vi "EventFinderV1.vi"() -> ()   [LabVIEW 2013]
uses:
  <vilib>/Analysis/baseanly.llb/Mean (DBL).vi
  <vilib>/Analysis/5stat.llb/RMS (DBL).vi
  <vilib>/Utility/file.llb/Write To Spreadsheet File (DBL).vi
  <vilib>/Analysis/NI_AALPro.lvlib
  <vilib>/Analysis/NI_AALBase.lvlib
panel:
  in  "Points":i32=2
  in  "Median filter":bool
  in  "Reverse trace in time":bool
  in  "Reduce points to display by factor":i32=10
  out "?":bool=TRUE
  in  "Peak over DNA level/nA":dbl=-0.05
  out "?":bool=TRUE
  in  "DNA level/nA":dbl=-0.1
  out "?":bool=TRUE
  in  "21 over DNA level/nA":dbl=-0.02
  in  "Each event as separate file":bool
  in  "Custom dt":cluster{"Custom dt":dbl, "Custom dt":bool}={"Custom dt"=4e-06, "Custom dt"=FALSE}
  in  "Fraction from start":dbl=0.1
  in  "Type 21 limit":bool
  in  "Baseline correction":T1={"Baseline correction?"=TRUE, "Correction method"=enum."Median", "Points for \nbaseline "=125000, "Value  if \nsubtracting"=0.0, "Order if using polynomial"=3, "Use file \nlength"=TRUE}
  in  "Output folder name":string="Output"
  in  "Loop over \nfolder of folders":bool
  in  "Directory of subfolders":path=path "F:/"
  out "Cumulative time/s":dbl=1130.5142
  out "File mean":dbl=-0.4359130217142997 format="%0.2f"
  out "File RMS":dbl=12.404886152154484 format="%0.4f"
  out "Cumulative time/s":dbl=1429.5900000000001
  in  "Numbers off":bool
  in  "Move this file to \n\"noise\" folder":bool
  in  "Graphs off":bool
  in  "Limit in peak current":bool
  in  "Invert trace":bool
  in  "Event begin+end/nA":dbl=-0.06
  in  "Each event in separate column":bool
  in  "Events concatenated into one column":bool
  in  "More than/fAs":dbl=50.0
  in  "Less than/fAs":dbl=500.0
  in  "Limit in area":bool
  out "Raw current":waveform(dbl)(graph)={"t0"=timestamp(0 s since 1904-01-01), "dt"=0.0002, "Y"=[]}
  in  "Pause at new file?":bool
  in  "Finish here":bool
  in  "Jump file":bool
  out "Time since last/s":dbl=0.2605 format="%0.5f"
  out "Time in file/s":dbl=0.9242 format="%0.3f"
  in  "Reject on":bool
  out "Duration/s":dbl=0.0009600000000000003 format="%0.5f"
  out "Mean current/nA":dbl=-108.25728329022725 format="%0.5f"
  out "Peak value/nA":dbl=-147.76609802246094 format="%0.5f"
  out "Event area/fAs":dbl=103839.10133361818 format="%0.5f"
  out "dt/s":dbl=2e-05
  in  "Event statistics":bool=TRUE
  out "Accepted events":i32=475
  in  "Reject":bool
  in  "Loop delay/s":dbl
  out "Current file":i32=5
  out "Current file name":path
  out "No files":i32=7
  in  "Directory of files":path=path "C:/"
  out "Event detection trace":waveform(dbl)(graph)={"t0"=timestamp(0 s since 1904-01-01), "dt"=2e-05, "Y"=[]}
  in  "Accept on":bool
  out "Current trace after filter, baseline correction":waveform(dbl)(graph)={"t0"=timestamp(0 s since 1904-01-01), "dt"=0.0002, "Y"=[]}
  in  "Accept":bool
  in  "Points before/after":i32=50
  in  "Min duration/s":dbl=0.0005
  in  "Threshold/nA":dbl=-0.1
  # "Event detection settings"
  # "Files to save"
  # "Data input settings"
  # "Limit in event area"
  # "Event stats"
  # "Speed up\n analysis"
  # "Slow analysis \nfor viewing"
  # "Actions"
  # "Further data input settings"
  # "Limit according to DNA level"
  # "Set DNA level:"
  # "Use files in multiple folders"
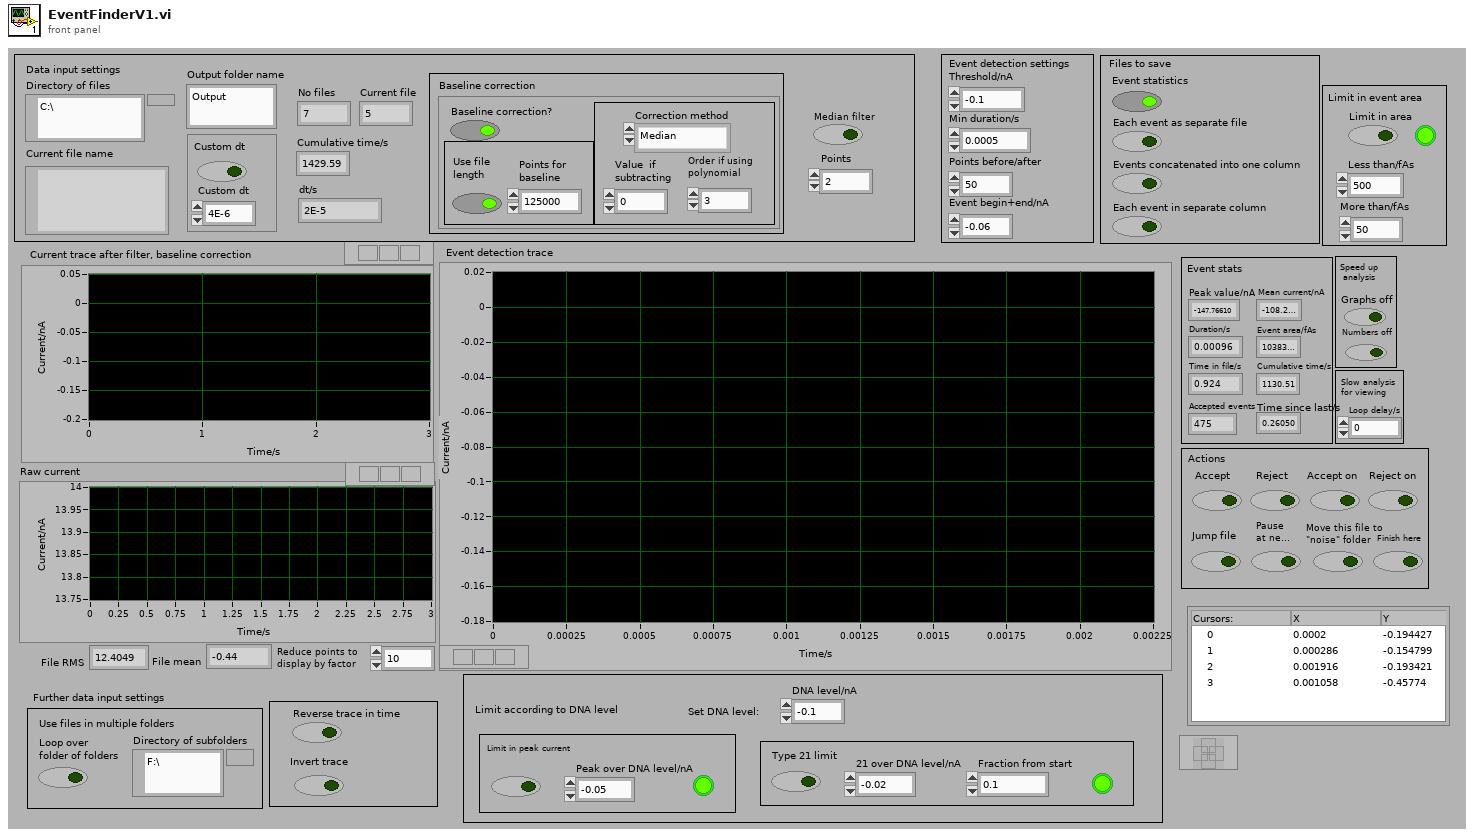
[diagram p1: front panel]
types:
  T1 = cluster{"Baseline correction?":bool, "Correction method":enum16{"Linear", "Median", "Mean", "Polynomial", "Subtraction"}, "Points for \nbaseline ":i32, "Value  if \nsubtracting":dbl, "Order if using polynomial":i32, "Use file \nlength":bool}
  T2 = enum16{"Linear", "Median", "Mean", "Polynomial", "Subtraction"}
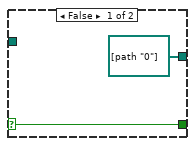
[diagram p2: hidden frame]
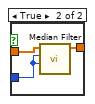
[diagram p7: hidden frame]
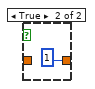
[diagram p8: hidden frame]
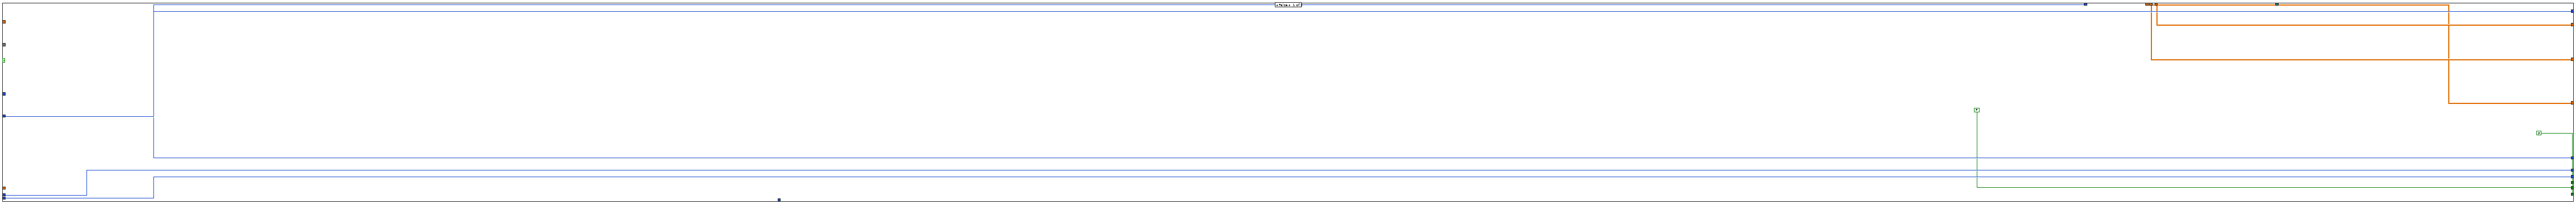
[diagram p15: hidden frame]
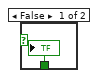
[diagram p18: hidden frame]
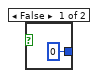
[diagram p20: hidden frame]
diagram:
  n1 = case shown="True" "Loop over \nfolder of folders" {
    selector: "Loop over \nfolder of folders" -> [w5 w7]
    tunnel: "Directory of subfolders" -> [_ w10]
    tunnel: [path[] [path "0"] w9] -> w4
    tunnel: [w5 w7] -> w3
    frame False {
    }
    frame True {
      n2 = List Folder(path=w10) -> (folder names=w8:string[])  [unwired: 1 in, 5 out]
      n3 = for {
        tunnel: w10 -> [w13]
        tunnel: [w12] -> w9 mode=indexing
        tunnel: w8 -> [w11] mode=indexing
        n4 = Build Path(base path=w13, name or relative path=w11) -> (appended path=w12:path)
      }
    }
  }
  n5 = for {
    tunnel: w4 -> [w33] mode=indexing
    tunnel: w3 -> [w21]
    # "Initialize arrays"
    # "Loop over folders if selected"
    n6 = case shown="False" w21 {
      tunnel: ["Directory of files" w72] -> w69
      tunnel: w33 -> [_ w72]
      frame False {
      }
      frame True {
      }
    }
    n7 = Initialize Array(0.0 ("element"), 0 ("dimension size"), 0 ("dimension size")) -> (w58:dbl[][])
    n8 = call "Make output folder.vi"("Output folder name"="Output folder name", "Folder"=w69) -> ("created path"=w68:path)
    n9 = call "Create array of files in folder.vi"("Folder"=w69) -> ("No files"=→"No files":i32, "Array of files in folder"=w14:path[])  [unwired: 1 in]
    n10 = Initialize Array(0.0 ("element"), 0 ("dimension size"), 0 ("dimension size")) -> (w53:dbl[][])
    n11 = Initialize Array(0.0 ("element"), 0 ("dimension size"), 0 ("dimension size")) -> (w64:dbl[][])
    n12 = for {
      tunnel: w14 -> [w101] mode=indexing
      tunnel: w68 -> [w99]
      shift-right: [w125] -> w36
      shift-left: w64 -> [w130]
      tunnel: [w91] -> w44
      shift-right: [w128] -> _
      shift-left: 0 -> [w129]
      shift-right: [w120] -> w57
      shift-left: w58 -> [w121]
      shift-right: [w118] -> w42
      shift-left: w53 -> [w119]
      shift-right: [w105] -> w28
      shift-left: 0 -> [w113]
      shift-right: [w106] -> _
      shift-left: 0.0 -> [w107]
      i -> [w131]
      stop <- w124 stop-if-true
      # "Loop over files in folder"
      n13 = Increment(x=w131) -> (x+1=w122:i32)
      "Current file" <- w122
      n14 = case shown="True" "Pause at new file?" {
        frame False {
        }
        frame True {
          n15 = property on="Reject on" class="Bool (strict)"("Value"=FALSE ("Keep rejecting")) -> ()  [unwired: 2 in, 2 out]
          n16 = property on="Accept on" class="Bool (strict)"("Value"=FALSE ("Keep accepting")) -> ()  [unwired: 2 in, 2 out]
        }
      }
      n17 = call "Baselinecorrector.vi"("Custom dt"="Custom dt", "Path"=w101, "Baseline param"="Baseline correction") -> ("Raw current"=w103:waveform(dbl), "Filtered, baseline corrected"=w89:dbl[], "dt"=w92:dbl)  [unwired: 3 in, 1 out]
      n18 = case shown="False" "Median filter" {
        tunnel: w89 -> [w133 w136]
        tunnel: "Points" -> [_ w135]
        tunnel: [w133 w134] -> w87
        frame False {
        }
        frame True {
          n19 = call <vilib>:"Median Filter.vi"("right rank"=w135, "left rank"=w135, "X"=w136) -> ("Filtered X"=w134:dbl[])  [unwired: 7 in, 1 out]
        }
      }
      n20 = case shown="True" "Reverse trace in time" {
        tunnel: w87 -> [w142 w144]
        tunnel: [w142 w143] -> w117
        frame False {
        }
        frame True {
          n21 = Reverse 1D Array(array=w144) -> (reversed array=w143:dbl[])
        }
      }
      n22 = case shown="True" "Invert trace" {
        tunnel: w117 -> [w139 w141]
        tunnel: [w139 w140] -> w102
        frame False {
        }
        frame True {
          n23 = Negate(x=w141) -> (-x=w140:dbl[])
        }
      }
      n24 = Array Size(array=w102) -> (size(s)=w97:i32)
      n25 = Add(x=w97, y=w113) -> (x+y=w112:i32)
      n26 = call-poly <vilib>:"Mean.vi"("X"=w102) -> ("mean"=→"File mean":dbl)  [unwired: 1 out]
      n27 = call-poly <vilib>:"RMS.vi"("X"=w102) -> ("rms value"=→"File RMS":dbl)  [unwired: 1 out]
      n28 = Bundle By Name("dt"=w92, "Y"=w102) -> (w114:waveform(dbl))  [unwired: 1 out]
      n29 = Equal To 0?(x=w92) -> (x = 0?=w110:bool)
      n30 = case shown="False" w110 {
        tunnel: [w137 1] -> w111
        tunnel: w92 -> [w137 _]
        frame False {
        }
        frame True {
        }
      }
      "dt/s" <- w111
      n31 = local read "Graphs off"() -> (w115:bool)
      n32 = call "Display traces.vi"("Graphs off"=w115, "Raw current in"=w103, "Display reduction"="Reduce points to display by factor", "Waveform"=w114) -> ("Raw current out"=→"Raw current":waveform(dbl), "Baseline corrected current trace"=→"Current trace after filter, baseline correction":waveform(dbl))  [unwired: 6 in]
      n33 = while {
        tunnel: w102 -> [w178]
        shift-right: [w180] -> _
        shift-left: 0 -> [w181]
        tunnel: w111 -> [w149]
        tunnel: w97 -> [w147]
        shift-right: [w166] -> w125
        shift-left: w130 -> [w177]
        shift-right: [w154] -> w128
        shift-left: w129 -> [w176]
        shift-right: [w175] -> _
        shift-left: 0 -> [w174]
        shift-right: [w171] -> _
        shift-left: 0 -> [w172]
        tunnel: [w167] -> w124
        tunnel: w122 -> [w165]
        shift-right: [w164] -> w120
        shift-left: w121 -> [w163]
        shift-right: [w161] -> w118
        shift-left: w119 -> [w162]
        tunnel: w112 -> [w153]
        tunnel: [w153] -> w105
        tunnel: w107 -> [w152]
        tunnel: [w149] -> w104
        tunnel: w99 -> [w148]
        tunnel: [w148] -> w91
        stop <- w168 stop-if-true
        # "While loop through file to search for events"
        n34 = Greater Or Equal?(x=w181, y=w147) -> (x >= y?=w169:bool)
        n35 = Increment(x=w181) -> (x+1=w179:i32)
        n36 = Index Array(array=w178, index=w179) -> (element=w160:dbl)
        n37 = Less?(x=w160, y="Threshold/nA") -> (x < y?=w159:bool)
        n38 = Multiply(x=w153, y=w149) -> (x*y=→"Cumulative time/s":dbl)
        n39 = case shown="True" w159 {
          tunnel: w178 -> [_ w249]
          tunnel: w179 -> [w203 w212]
          tunnel: [w203 w221] -> w180
          tunnel: "Points before/after" -> [_ w220]
          tunnel: w149 -> [_ w214]
          tunnel: [w202 w245] -> w166
          tunnel: w177 -> [w202 w215]
          tunnel: w176 -> [w201 w244]
          tunnel: [w201 w243] -> w154
          tunnel: [w200 w242] -> w175
          tunnel: w174 -> [w200 w207]
          tunnel: w172 -> [w199 w237]
          tunnel: [w199 w238] -> w171
          tunnel: [w195 w236] -> w170
          tunnel: [FALSE ("Finish here") w235] -> w167
          tunnel: w165 -> [_ w234]
          tunnel: w163 -> [w197 w233]
          tunnel: [w197 w232] -> w164
          tunnel: w162 -> [w196 w231]
          tunnel: [w196 w230] -> w161
          tunnel: [w195 w229] -> w156
          tunnel: w152 -> [_ w213]
          tunnel: w148 -> [_ w224]
          frame False {
            w195 = FALSE
          }
          frame True {
            n40 = call "Index of first cross.vi"(">Index of threshold cross>"=w212, ">y>"=w249, "Event begin+end/nA"="Event begin+end/nA") -> ("Numeric"=w222:i32)  [unwired: 8 in]
            n41 = call "Event end index.vi"(">Index of threshold cross>"=w212, ">y>"=w249, "Event begin+end/nA"="Event begin+end/nA") -> ("Numeric"=w221:i32)  [unwired: 8 in]
            n42 = formula code="int a;\nint b;\nint c;\nfloat d;\nfloat e;\nfloat f;\nfloat g;\nfloat h;\na=start-points;\nb=2*points+(end-start);\nc=end-start;\nd=index*dt;\ne=d+time;\nf=points*dt;\ng=(c+points)*dt;\nh=(index-ok)*dt;"("start"=w222, "end"=w221, "points"=w220, "dt"=w214, "time"=w213, "index"=w212, "ok"=w207) -> ("a"=w219:i32, "b"=w218:i32, "d"=w211:dbl, "e"=w210:dbl, "f"=w209:dbl, "g"=w208:dbl, "h"=w205:dbl)  [unwired: 1 out]
            n43 = Array Subset(array=w249, index=w219, length=w218) -> (w216:dbl[])
            n44 = local read "Graphs off"() -> (w204:bool)
            n45 = Bundle By Name("dt"=w214, "Y"=w216) -> (w227:waveform(dbl))  [unwired: 1 out]
            n46 = case shown="False" w204 {
              tunnel: w227 -> [w350 _]
              frame False {
                "Event detection trace" <- w350
              }
              frame True {
              }
            }
            n47 = local read "Numbers off"() -> (w217:bool)
            n48 = case shown="False" w217 {
              tunnel: w211 -> [w351 _]
              frame False {
                "Time in file/s" <- w351
              }
              frame True {
              }
            }
            n49 = case shown="False" w217 {
              tunnel: w205 -> [w349 _]
              tunnel: w210 -> [w348 _]
              frame False {
                "Time since last/s" <- w349
                "Cumulative time/s" <- w348
              }
              frame True {
              }
            }
            n50 = control-ref of="Event detection trace"() -> (w206:refnum<vi>)
            n51 = local read "Graphs off"() -> (w226:bool)
            n52 = call "Display cursors.vi"("Numeric"=w208, "Graphs off"=w226, "Numeric 2"=w209, "Fraction from start"="Fraction from start", "WaveformGraph in"=w206) -> ()  [unwired: 7 in]
            n53 = while {
              tunnel: [w301] -> w240
              tunnel: [w307] -> w241
              tunnel: [w260] -> w248
              tunnel: w205 -> [w304]
              tunnel: w237 -> [w303]
              tunnel: [w303] -> w239
              tunnel: w211 -> [w250]
              tunnel: w216 -> [w286]
              tunnel: w214 -> [w289]
              tunnel: [w296] -> w236
              tunnel: [w299] -> w235
              tunnel: w234 -> [w263]
              tunnel: w209 -> [w294]
              tunnel: w208 -> [w290]
              tunnel: [w295] -> w229
              tunnel: w210 -> [w261]
              tunnel: [w289] -> w225
              tunnel: "Fraction from start" -> [w287]
              stop <- w300 stop-if-true
              n54 = Equal?(x=0, y=w303) -> (x = y?=w305:bool)
              n55 = case shown="False" w305 {
                tunnel: w304 -> [w346 _]
                tunnel: [w346 nan] -> w264
                frame False {
                }
                frame True {
                }
              }
              n56 = call "Cursoreventanalysis.vi"("Input array"=w286, "dt"=w289, "Cursor 1"=w294, "Cursor 2"=w290) -> ("Event area/fAs"=w265:dbl, "Peak current value/nA"=w266:dbl, "Mean event current/nA"=w267:dbl, "Event duration/s"=w268:dbl, "Statistics array"=w262:dbl[])  [unwired: 7 out]
              n57 = Build Array (concatenate)(w262, w264, w250, w263, w261) -> (w257:dbl[])
              n58 = local read "Numbers off"() -> (w288:bool)
              n59 = Multiply(x="Loop delay/s", y=1000.0) -> (x*y=w274:dbl)
              n60 = case shown="False" w288 {
                tunnel: w267 -> [w343 _]
                tunnel: w268 -> [w342 _]
                tunnel: w265 -> [w341 _]
                tunnel: w266 -> [w340 _]
                frame False {
                  "Event area/fAs" <- w341
                  "Peak value/nA" <- w340
                  "Mean current/nA" <- w343
                  "Duration/s" <- w342
                }
                frame True {
                }
              }
              n61 = Wait (ms)(milliseconds to wait=w274) -> ()  [unwired: 1 out]
              n62 = property on="Raw current" class="WFGraph (strict)"("Cursor.Cursor X"=w250, "Active Cursor"=u32 1) -> ()  [unwired: 2 in, 2 out]
              n63 = property on="Current trace after filter, baseline correction" class="WFGraph (strict)"("Cursor.Cursor X"=w250, "Active Cursor"=u32 0) -> ()  [unwired: 2 in, 2 out]
              n64 = Add(x="DNA level/nA", y="21 over DNA level/nA") -> (x+y=w254:dbl)
              n65 = Divide(x=w294, y=w289) -> (x/y=w293:dbl)
              n66 = call "Type21 test.vi"("Type 21 limit"="Type 21 limit", "Event duration/s"=w268, ">dt>"=w289, ">Detected event array>"=w286, "Numeric 2"=w293, "Fraction from start"=w287, "Numeric"=w254) -> ("Boolean"=w269:bool, "Boolean 2"=w282:bool)  [unwired: 3 in]
              n67 = case shown="True" w282 {
                tunnel: [0 1] -> w256
                frame False {
                }
                frame True {
                }
              }
              n68 = local read "Numbers off"() -> (w271:bool)
              n69 = Build Array (concatenate)(w257, w256) -> (w255:dbl[])
              n70 = case shown="False" w271 {
                tunnel: w282 -> [w332 _]
                frame False {
                  "?" <- w332
                }
                frame True {
                }
              }
              n71 = Add(x="Peak over DNA level/nA", y="DNA level/nA") -> (x+y=w284:dbl)
              n72 = local read "Numbers off"() -> (w270:bool)
              n73 = Greater?(x=w284, y=w266) -> (0:w283:bool)
              n74 = case shown="False" w270 {
                tunnel: w283 -> [w331 _]
                frame False {
                  "?" <- w331
                }
                frame True {
                }
              }
              n75 = case shown="False" w283 {
                tunnel: [0 1] -> w258
                frame False {
                }
                frame True {
                }
              }
              n76 = Build Array (concatenate)(w255, w258) -> (w260:dbl[])
              n77 = case shown="False" "Limit in peak current" {
                tunnel: w266 -> [_ _]
                tunnel: w266 -> [_ _]
                tunnel: [FALSE w345] -> w291
                tunnel: w283 -> [_ w345]
                frame False {
                }
                frame True {
                }
              }
              n78 = Greater?(x="More than/fAs", y=w265) -> (0:w278:bool)
              n79 = Less?(x="Less than/fAs", y=w265) -> (x < y?=w279:bool)
              n80 = local read "Numbers off"() -> (w272:bool)
              n81 = Or(x=w278, y=w279) -> (x .or. y?=w276:bool)
              n82 = case shown="False" "Limit in area" {
                tunnel: [FALSE w335] -> w275
                tunnel: w276 -> [_ w335]
                frame False {
                }
                frame True {
                }
              }
              n83 = case shown="True" w272 {
                tunnel: w276 -> [w333 _]
                frame False {
                  "?" <- w333
                }
                frame True {
                }
              }
              n84 = Less?(x=w268, y="Min duration/s") -> (x < y?=w298:bool)
              n85 = flat-sequence {
                tunnel: [w328] -> w307
                tunnel: [w324] -> w301
                tunnel: [w320] -> w300
                tunnel: ["Finish here"] -> w299
                tunnel: w298 -> [w318]
                tunnel: [w314] -> w296
                tunnel: ["Move this file to \n\"noise\" folder"] -> w295
                tunnel: w291 -> [w311]
                tunnel: w275 -> [w310]
                tunnel: w269 -> [w309]
                frame #0 {
                  n86 = Or(x="Accept", y="Accept on") -> (x .or. y?=w328:bool)
                  n87 = Or(x="Reject", y="Reject on") -> (x .or. y?=w323:bool)
                  n88 = Or(x=w311, y=w309) -> (x .or. y?=w312:bool)
                  n89 = Or(x=w318, y=w310) -> (x .or. y?=w317:bool)
                  n90 = Or(x=w317, y=w312) -> (x .or. y?=w316:bool)
                  n91 = Or(x=w323, y=w328) -> (x .or. y?=w325:bool)
                  n92 = Or(x=w316, y=w323) -> (x .or. y?=w324:bool)
                  n93 = Or(x=w316, y=w325) -> (x .or. y?=w322:bool)
                  n94 = Or(x="Jump file", y="Move this file to \n\"noise\" folder") -> (x .or. y?=w314:bool)
                  n95 = Or(x=w314, y=w322) -> (x .or. y?=w321:bool)
                  n96 = Or(x=w321, y="Finish here") -> (x .or. y?=w320:bool)
                }
              }
            }
            n97 = Not(x=w240) -> (.not. x?=w247:bool)
            n98 = And(x=w247, y=w241) -> (x .and. y?=w246:bool)
            n99 = case shown="True" w246 {
              tunnel: w215 -> [w357 w375]
              tunnel: w248 -> [_ w374]
              tunnel: [w357 w373] -> w245
              tunnel: w244 -> [w356 w372]
              tunnel: [w356 w358] -> w243
              tunnel: w207 -> [w355 _]
              tunnel: w212 -> [_ w361]
              tunnel: [w355 w361] -> w242
              tunnel: w239 -> [w354 w371]
              tunnel: [w354 w370] -> w238
              tunnel: w216 -> [_ w363]
              tunnel: w233 -> [w353 w369]
              tunnel: [w353 w368] -> w232
              tunnel: w231 -> [w352 w367]
              tunnel: [w352 w366] -> w230
              tunnel: w225 -> [_ w360]
              tunnel: w224 -> [_ w359]
              frame False {
              }
              frame True {
                n100 = Increment(x=w371) -> (x+1=w370:i32)
                n101 = Increment(x=w372) -> (x+1=w358:i32)
                n102 = Insert Into Array(array=w375, new element=w374) -> (w373:dbl[][])  [unwired: 2 in]
                n103 = case shown="True" "Each event in separate column" {
                  tunnel: w369 -> [w376 w379]
                  tunnel: [w376 w378] -> w368
                  tunnel: w363 -> [_ w377]
                  frame False {
                  }
                  frame True {
                    n104 = Insert Into Array(array=w379, index (row)=0, new element=w377) -> (w378:dbl[][])  [unwired: 1 in]
                  }
                }
                n105 = call "Concatenated events.vi"("dt"=w360, "Array 3"=w367, "Events concatenated into one column"="Events concatenated into one column", "Array in"=w363) -> ("Array out"=w366:dbl[][])  [unwired: 7 in]
                n106 = call "Save separate events.vi"("dt"=w360, "Each event as separate file"="Each event as separate file", "Array"=w363, "Numeric"=w358, "created path"=w359) -> ()  [unwired: 7 in]
              }
            }
          }
        }
        n107 = Or(x=w170, y=w169) -> (x .or. y?=w158:bool)
        n108 = Or(x=w156, y=w158) -> (x .or. y?=w157:bool)
        n109 = case shown="True" w156 {
          frame False {
          }
          frame True {
            n110 = flat-sequence {
              tunnel: [w184] -> w183
              tunnel: w183 -> [w193]
              frame #0 {
                n111 = local read "Directory of files"() -> (w185:path)
                n112 = Build Path(base path=w185, name or relative path="Noise") -> (appended path=w188:path)
                n113 = call <vilib>:"Check if File or Folder Exists.vi"("path"=w188) -> ("file or folder exists?"=w187:bool, "dup path"=w186:path)  [unwired: 1 in, 8 out]
                n114 = case shown="False" w187 {
                  tunnel: w186 -> [w190 w192]
                  tunnel: [w191 w192] -> w184
                  frame False {
                    n115 = Create Folder(path (use dialog)=w190) -> (created path=w191:path)  [unwired: 1 in, 3 out]
                  }
                  frame True {
                  }
                }
              }
              frame #1 {
                n116 = local read "Current file name"() -> (w194:path)
                n117 = Move(source path=w194, 10:w193) -> ()  [unwired: 1 in, 5 out]
              }
            }
          }
        }
        n118 = Or(x=w157, y=w167) -> (x .or. y?=w168:bool)
        n119 = local read "Numbers off"() -> (w155:bool)
        n120 = case shown="False" w155 {
          tunnel: w154 -> [w182 _]
          frame False {
            "Accepted events" <- w182
          }
          frame True {
          }
        }
      }
      n121 = Multiply(x=w104, y=w105) -> (x*y=w106:dbl)
      "Current file name" <- w101
    }
    n122 = local read "Events concatenated into one column"() -> (w52:bool)
    n123 = local read "Each event in separate column"() -> (w51:bool)
    n124 = Index Array(array=w36, index (col)=7 ("disabled index (col)")) -> (element=w37:dbl[])  [unwired: 1 in]
    n125 = case shown="True" w52 {
      tunnel: w44 -> [_ w81]
      tunnel: w42 -> [_ w79]
      frame False {
      }
      frame True {
        n126 = call "Save 2D data as tdms.vi"("Array"=w79, "String to add"="Timed events", "created path"=w81) -> ()  [unwired: 9 in]
      }
    }
    n127 = case shown="True" w51 {
      tunnel: w44 -> [_ w83]
      tunnel: w57 -> [_ w84]
      frame False {
      }
      frame True {
        n128 = call "Save 2D data as tdms.vi"("Array"=w84, "String to add"="Multicolumn", "created path"=w83) -> ()  [unwired: 9 in]
      }
    }
    n129 = Array Size(array=w37) -> (size(s)=w25:i32)
    n130 = for {
      N: w25 -> [_]
      tunnel: w37 -> [w74]
      tunnel: [w73] -> w34 mode=indexing
      i -> [w78]
      n131 = Index Array(array=w74, index=w78) -> (element=w76:dbl)
      n132 = Decrement(x=w78) -> (x-1=w77:i32)
      n133 = Index Array(array=w74, index=w77) -> (element=w75:dbl)
      n134 = Subtract(x=w76, y=w75) -> (x-y=w73:dbl)
    }
    n135 = local read "dt/s"() -> (w27:dbl)
    n136 = Multiply(x=w28, y=w27) -> (x*y=w26:dbl)
    n137 = Insert Into Array(array=w36, index (col)=8 ("disabled index (col)"), new element=w34) -> (w30:dbl[][])  [unwired: 1 in]
    n138 = for {
      N: w25 -> [_]
      tunnel: w26 -> [w70]
      tunnel: [w70] -> w24 mode=indexing
    }
    n139 = Insert Into Array(array=w30, index (col)=9 ("disabled index (col)"), new element=w24) -> (w29:dbl[][])  [unwired: 1 in]
    n140 = case shown="True" "Event statistics" {
      tunnel: w44 -> [_ w86]
      tunnel: w29 -> [_ w85]
      frame False {
      }
      frame True {
        n141 = call "Saveeventstatistics.vi"("created path"=w86, "Array"=w85) -> ()  [unwired: 10 in]
      }
    }
    n142 = local read "Threshold/nA"() -> (w47:dbl)
    n143 = local read "Baseline correction"() -> (w19:T1)
    n144 = call "Save event stats.vi"("created path"=w44) -> ("Path"=w48:path)  [unwired: 10 in]
    n145 = local read "Min duration/s"() -> (w46:dbl)
    n146 = local read "Points before/after"() -> (w16:i32)
    n147 = local read "dt/s"() -> (w40:dbl)
    n148 = local read "Less than/fAs"() -> (w23:dbl)
    n149 = local read "More than/fAs"() -> (w22:dbl)
    n150 = local read "Event begin+end/nA"() -> (w15:dbl)
    n151 = Unbundle(w19) -> ("Correction method"=w17:T2, "Points for \nbaseline"=w18:i32)  [unwired: 4 out]
    n152 = Multiply(x=w28, y=w40) -> (x*y=w39:dbl)
    n153 = Build Array(w47, w46, w18, w17, w28, w39, w23, w22, w16, w15) -> (w45:dbl[])
    n154 = call-poly <vilib>:"Write To Spreadsheet File.vi"("format (%.3f)"="%.6f", "append to file? (new file:F)"=TRUE, "1D data"=w45, "file path (dialog if empty)"=w48) -> ()  [unwired: 4 in, 1 out]
  }
